vi "get wait ring.vi"(8 "error in (no error)":errorcluster caption="에러 입력(에러 없음)", 11 "DW7912 입력":refnum<class "DW7912.lvclass">) -> (0 "error out":errorcluster caption="에러 출력", 1 "caption":string="Wait", 2 "strings & values":T1=[{"String"="0us", "Value"=0}, {"String"="166us", "Value"=1}, {"String"="332us", "Value"=2}, {"String"="498us", "Value"=3}, {"String"="664us", "Value"=4}, {"String"="830us", "Value"=5}, {"String"="996us", "Value"=6}, {"String"="1162us", "Value"=7}, {"String"="1328us", "Value"=8}, {"String"="1494us", "Value"=9}, {"String"="1660us", "Value"=10}, {"String"="1826us", "Value"=11}, {"String"="1992us", "Value"=12}, {"String"="2158us", "Value"=13}, {"String"="2324us", "Value"=14}, {"String"="2490us", "Value"=15}], 3 "DW7912 출력":refnum<class "DW7912.lvclass">, 4 "default value":u8, 6 "using":bool=TRUE)   [LabVIEW 2020, in "DW7912.lvclass"]
uses:
  DW7912.lvclass
  <vilib>/Utility/miscctls.llb/LVStringsAndValuesArrayTypeDef_U8.ctl
  Haptic IC/Haptic IC.lvclass
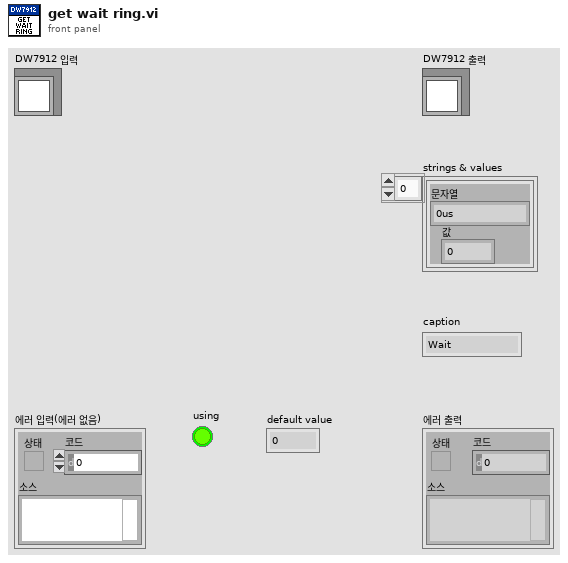
[diagram p1: front panel]
types:
  T1 = typedef "LVStringsAndValuesArrayTypeDef_U8.ctl" = cluster{"String":string, "Value":u8}[]
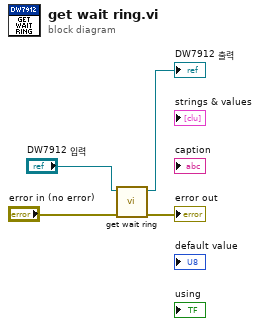
[diagram p0: block diagram]
diagram:
  n1 = call-parent "get wait ring.vi"("error in (no error)"="error in (no error)", "Haptic IC 입력"="DW7912 입력") -> ("error out"=→"error out":errorcluster, "Haptic IC 출력"=→"DW7912 출력":refnum<class "DW7912.lvclass">)  [unwired: 4 in, 4 out]
